vi "FVI_Swerve_offset direction.vi"(9 "Correction angle":dbl, 11 "SwerveDrive in":T1) -> (3 "SwerveDrive out":T1)   [LabVIEW 2018]
uses:
  SwerveDrive.ctl
  <vilib>/Analysis/coordinate.llb/Angle Units.ctl
  <vilib>/Analysis/coordinate.llb/Angle Range (Degree).ctl
  <vilib>/Analysis/coordinate.llb/Wrap Angle (array).vi
  <vilib>/Analysis/NI_AAL_Angle.lvlib
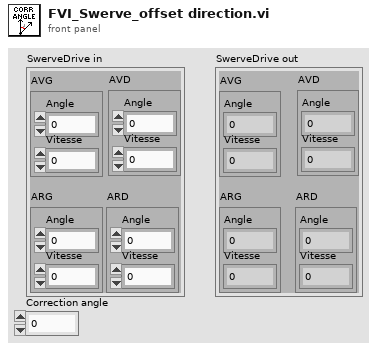
[diagram p1: front panel]
types:
  T1 = typedef "SwerveDrive.ctl" = cluster{"AVD":cluster{"Angle":dbl, "Vitesse":dbl}, "AVG":cluster{"Angle":dbl, "Vitesse":dbl}, "ARG":cluster{"Angle":dbl, "Vitesse":dbl}, "ARD":cluster{"Angle":dbl, "Vitesse":dbl}}
  T2 = typedef "NI_AAL_Angle.lvlib/Angle Range (Degree).ctl" = u16
  T3 = typedef "NI_AAL_Angle.lvlib/Angle Units.ctl" = i32
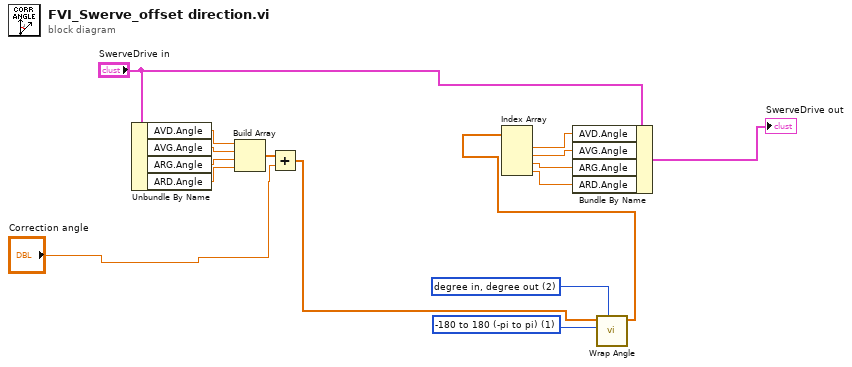
[diagram p0: block diagram]
diagram:
  w8 = T2 1 items=["none", "-180 to 180 (-pi to pi)", "0 to 360 (0 to 2pi)"] ("angle range")
  w9 = T3 2 items=["radian in, radian out", "radian in, degree out", "degree in, degree out", "degree in, radian out"] ("angle units")
  n1 = Unbundle By Name("SwerveDrive in") -> ("AVD.Angle"=w11:dbl, "AVG.Angle"=w14:dbl, "ARG.Angle"=w13:dbl, "ARD.Angle"=w12:dbl)
  n2 = Build Array(w11, w14, w13, w12) -> (w10:dbl[])
  n3 = Add(x=w10, y="Correction angle") -> (x+y=w7:dbl[])
  n4 = call-poly <vilib>:"Wrap Angle.vi"("angle units"=w9, "angle range"=w8, "Angle In"=w7) -> ("Angle Out"=w2:dbl[])  [unwired: 7 in, 1 out]
  n5 = Index Array(array=w2) -> (element #1=w6:dbl, element #2=w5:dbl, element #3=w4:dbl, element #4=w3:dbl)  [unwired: 4 in]
  n6 = Bundle By Name(cluster="SwerveDrive in", "AVD.Angle"=w6, "AVG.Angle"=w5, "ARG.Angle"=w4, "ARD.Angle"=w3) -> (→"SwerveDrive out":T1)
